vi "svfa_Coerce M to Factor of N.vi"(2 "M":i32=1000, 3 "Block Size":i32=1000) -> (0 "Coerced M":i32, 1 "Zoom FFT Size":i32)   [LabVIEW 2017]
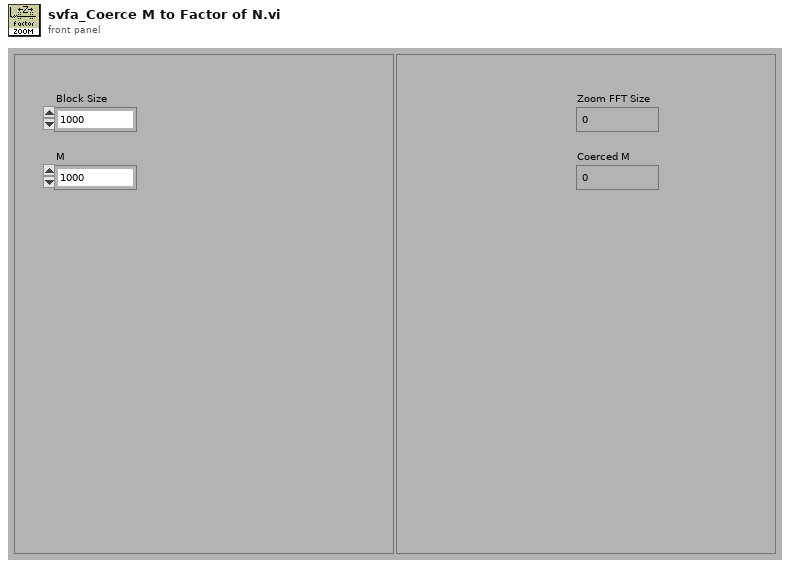
[diagram p1: front panel]
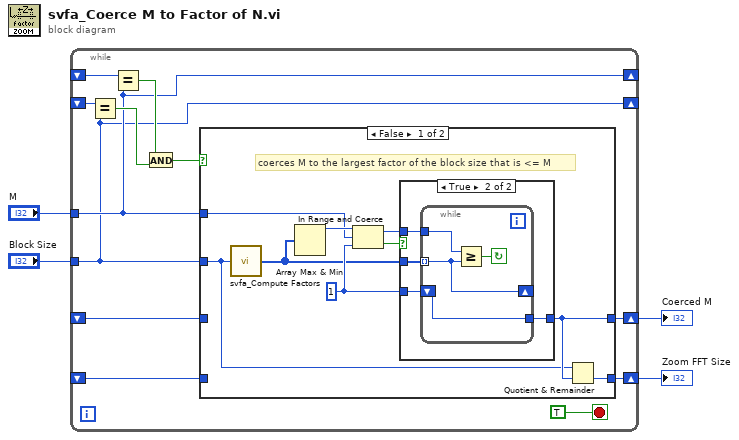
[diagram p0: block diagram]
diagram:
  n1 = while {
    shift-left: _ -> [w8]
    shift-right: [w10] -> w1
    shift-left: _ -> [w9]
    shift-right: [w11] -> w2
    shift-left: _ -> [w6]
    shift-right: [w5] -> _
    shift-left: _ -> [w15]
    shift-right: [w7] -> _
    tunnel: "Block Size" -> [w5]
    tunnel: "M" -> [w7]
    stop <- TRUE stop-if-true
    n2 = Equal?(x=w6, y=w5) -> (x = y?=w14:bool)
    n3 = Equal?(x=w15, y=w7) -> (x = y?=w13:bool)
    n4 = And(x=w13, y=w14) -> (x .and. y?=w12:bool)
    n5 = case shown="False" w12 {
      tunnel: w7 -> [w17 _]
      tunnel: [w23 w36] -> w11
      tunnel: w5 -> [w22 _]
      tunnel: [w21 w35] -> w10
      tunnel: w9 -> [_ w36]
      tunnel: w8 -> [_ w35]
      frame False {
        w20 = 1 ("lower limit")
        # "coerces M to the largest factor of the block size that is <= M"
        n6 = call <vilib>:"svfa_Compute Factors.vi"("Number to be factored"=w22) -> ("Factors of Input"=w19:i32[])
        n7 = Array Max & Min(array=w19) -> (max value=w18:i32)  [unwired: 3 out]
        n8 = In Range and Coerce(upper limit=w18, x=w17, lower limit=w20) -> (coerced(x)=w25:i32, In Range?=w24:bool)
        n9 = case shown="True" w24 {
          tunnel: [w26 w30] -> w23
          tunnel: w19 -> [_ w29]
          tunnel: w25 -> [w26 w28]
          tunnel: w20 -> [_ w27]
          frame False {
          }
          frame True {
            n10 = while {
              tunnel: [w31] -> w30
              shift-left: w27 -> [w31]
              shift-right: [w32] -> _
              tunnel: w28 -> [w33]
              tunnel: w29 -> [w32] mode=indexing
              stop <- w34 continue-if-true
              n11 = Greater Or Equal?(x=w33, y=w32) -> (x >= y?=w34:bool)
            }
          }
        }
        n12 = Quotient & Remainder(x=w22, y=w23) -> (floor(x/y)=w21:i32)  [unwired: 1 out]
      }
      frame True {
        # "inputs are the same as previous run --> pass the previous results"
      }
    }
  }
  "Coerced M" <- w2
  "Zoom FFT Size" <- w1
